vi "saveImage.vi"(8 "error in (no error)":errorcluster, 9 "I16bit image data":u16[][](array[numeric]), 10 "Path":path, 11 "Pixelfly in":refnum<class "Pixelfly.lvclass">) -> (0 "error out":errorcluster, 3 "Pixelfly out":refnum<class "Pixelfly.lvclass">)   [LabVIEW 2011, in "Hardware.lvlib" / "Channels.lvlib" / "Pixelfly.lvclass"]
uses:
  Pixelfly.lvclass
  Pixelfly.lvclass/Pixelfly.ctl
  Camera.lvclass
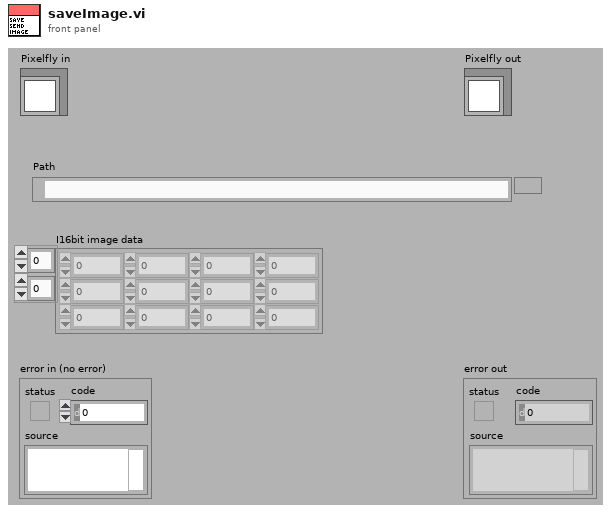
[diagram p1: front panel]
types:
  T1 = cluster{"cameraType":string, "imageName":string, "saved":string, "analysisType":string, "I16bit image data":u16[][], "path":path}
  T2 = typedef "Image Type" = u32
  T3 = typedef "IMAQ Image.ctl" = refnum<image>
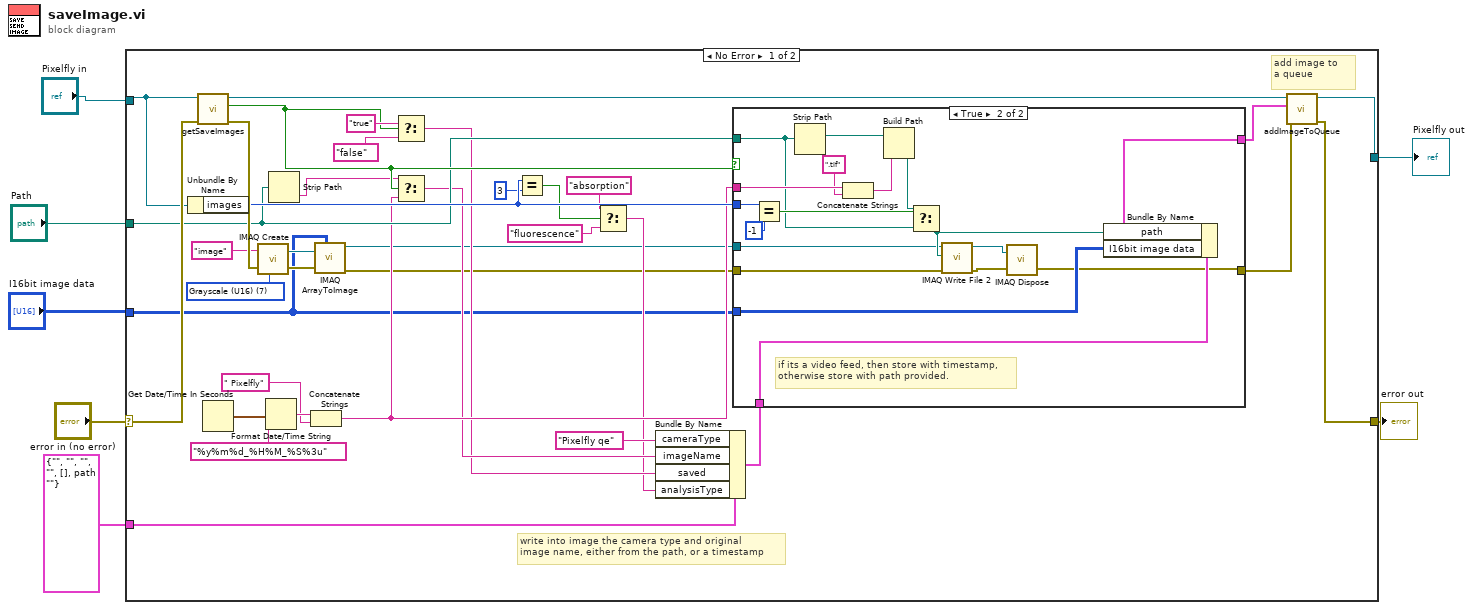
[diagram p0: block diagram]
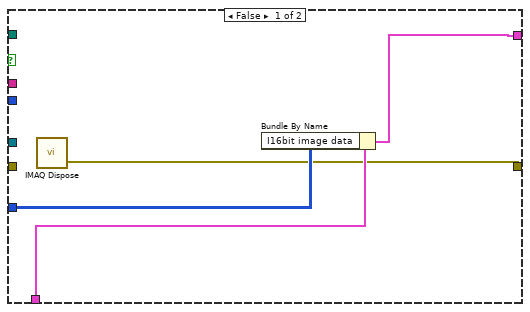
[diagram p2: hidden frame]
diagram:
  n1 = case shown="No Error" "error in (no error)" {
    selector: "error in (no error)" -> [w43 w67]
    tunnel: [w35 w67] -> w6
    tunnel: [w36 w66] -> w4
    tunnel: "Pixelfly in" -> [w27 w66]
    tunnel: "Path" -> [w20 _]
    tunnel: "I16bit image data" -> [w8 _]
    tunnel: T1 {"cameraType"="", "imageName"="", "saved"="", "analysisType"="", "I16bit image data"=[], "path"=path ""} ("ImageData") -> [w17 _]
    frame No Error {
      w40 = T2 7 items=["Grayscale (U8)", "Grayscale (I16)", "Grayscale (SGL)", "Complex (CSG)", "RGB (U32)", "HSL (U32)", "RGB (U64)", "Grayscale (U16)"] ("Image Type")
      # "write into image the camera type and original\nimage name, either from the path, or a timestamp"
      # "add image to\na queue"
      n2 = Unbundle By Name(w27) -> ("images"=w26:i32)
      n3 = call "getSaveImages.vi"("error in (no error)"=w43, "Camera in"=w27) -> ("error out"=w42:errorcluster, "saveImages?"=w21:bool, "Camera out"=w37:refnum<class "Pixelfly.lvclass">)  [unwired: 7 in]
      n4 = Get Date/Time In Seconds() -> (seconds since 1Jan1904=w34:timestamp)
      n5 = call "IMAQ Create"("Image Name"="image", "Image Type"=w40, "error in (no error)"=w42) -> ("New Image"=w39:T3, "error out"=w38:errorcluster)  [unwired: 2 in]
      n6 = Format Date/Time String(time format string (%c)="%y%m%d_%H%M_%S%3u", seconds (now)=w34) -> (date/time string=w32:string)  [unwired: 1 in]
      n7 = Strip Path(path=w20) -> (name=w19:string)  [unwired: 1 out]
      n8 = Concatenate Strings(w32, " Pixelfly") -> (w18:string)
      n9 = call "IMAQ ArrayToImage"("Image Pixels (U16)"=w8, "error in (no error)"=w38, "Image"=w39) -> ("error out"=w9:errorcluster, "Image Out"=w10:T3)  [unwired: 7 in]
      n10 = Select(t="true", s=w21, f="false") -> (s? t:f=w14:string)
      n11 = Select(t=w19, s=w21, f=w18) -> (s? t:f=w15:string)
      n12 = Equal?(x=w26, y=3) -> (x = y?=w24:bool)
      n13 = Select(t="absorption", s=w24, f="fluorescence") -> (s? t:f=w13:string)
      n14 = Bundle By Name(cluster=w17, "cameraType"="Pixelfly qe", "imageName"=w15, "saved"=w14, "analysisType"=w13) -> (w12:T1)
      n15 = case shown="True" w21 {
        tunnel: [w44 w51] -> w28
        tunnel: [w46 w55] -> w11
        tunnel: w20 -> [_ w57]
        tunnel: w18 -> [_ w64]
        tunnel: w26 -> [_ w61]
        tunnel: w12 -> [w47 w56]
        tunnel: w8 -> [w45 w53]
        tunnel: w10 -> [_ w49]
        tunnel: w9 -> [_ w48]
        frame False {
          n16 = call "IMAQ Dispose"() -> ("error out"=w44:errorcluster)  [unwired: 6 in]
          n17 = Bundle By Name(cluster=w47, "I16bit image data"=w45) -> (w46:T1)
        }
        frame True {
          # "if its a video feed, then store with timestamp,\notherwise store with path provided."
          n18 = Equal?(x=w61, y=-1) -> (x = y?=w58:bool)
          n19 = Strip Path(path=w57) -> (stripped path=w65:path)  [unwired: 1 out]
          n20 = Concatenate Strings(w64, ".tif") -> (w62:string)
          n21 = Build Path(base path=w65, name or relative path=w62) -> (appended path=w59:path)
          n22 = Select(t=w59, s=w58, f=w57) -> (s? t:f=w54:path)
          n23 = call-poly "IMAQ Write File 2"("error in (no error)"=w48, "File Path"=w54, "Image"=w49) -> ("error out"=w50:errorcluster, "Image Out (duplicate)"=w52:T3)  [unwired: 7 in]
          n24 = call "IMAQ Dispose"("Image"=w52, "error in (no error)"=w50) -> ("error out"=w51:errorcluster)  [unwired: 4 in]
          n25 = Bundle By Name(cluster=w56, "path"=w54, "I16bit image data"=w53) -> (w55:T1)
        }
      }
      n26 = call "addImageToQueue.vi"("error in (no error)"=w28, "ImageData"=w11, "Camera in"=w37) -> ("error out"=w35:errorcluster, "Camera out"=w36:refnum<class "Pixelfly.lvclass">)  [unwired: 7 in]
    }
    frame Error {
    }
  }
  "error out" <- w6
  "Pixelfly out" <- w4
